vi "Configure Timer Interval Error Filter.vi"(0 "VISA resource name":refnum<visa-resource-name>, 1 "Enable TIE Filter (F: Disable)":bool, 5 "TIE Filter Stopping Frequency (1.5E+6 Hz)":dbl=1500000.0, 7 "TIE Filter Starting Frequency (15000 Hz)":dbl=15000.0, 11 "error in (no error)":errorcluster) -> (4 "VISA resource name out":refnum<visa-resource-name>, 15 "error out":errorcluster)   [LabVIEW 2013, in "Agilent 90000 Series.lvlib"]
doc: "Configures the timer interval error filter characteristics."
uses:
  Agilent 90000 Series.lvlib
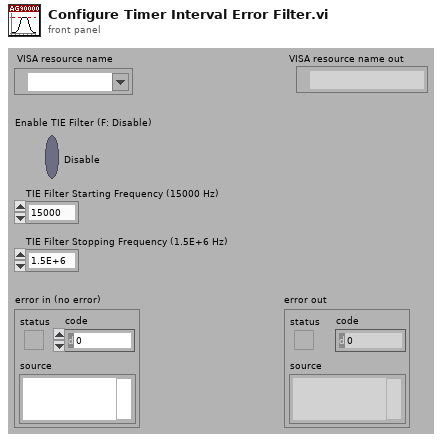
[diagram p1: front panel]
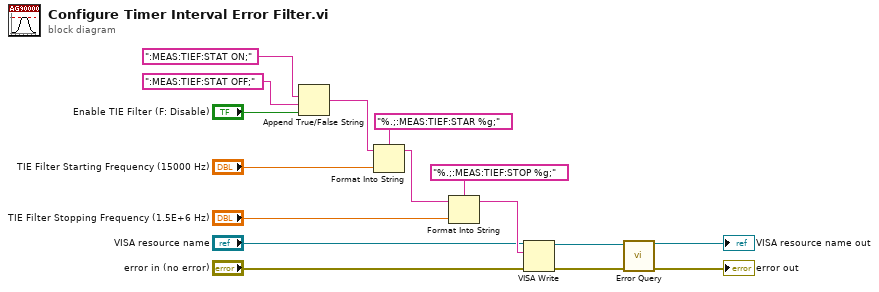
[diagram p0: block diagram]
diagram:
  n1 = Append True/False String(1:"Enable TIE Filter (F: Disable)", 2:":MEAS:TIEF:STAT OFF;", 3:":MEAS:TIEF:STAT ON;") -> (0:w13:string)  [unwired: 1 out]
  n2 = Format Into String(format string="%.;:MEAS:TIEF:STAR %g;", initial string=w13, "TIE Filter Starting Frequency (15000 Hz)") -> (resulting string=w10:string)  [unwired: 1 in, 1 out]
  n3 = Format Into String(format string="%.;:MEAS:TIEF:STOP %g;", initial string=w10, "TIE Filter Stopping Frequency (1.5E+6 Hz)") -> (resulting string=w7:string)  [unwired: 1 in, 1 out]
  n4 = VISA Write(VISA resource name="VISA resource name", write buffer=w7, error in (no error)="error in (no error)") -> (VISA resource name out=w4:refnum<visa-resource-name>, error out=w3:errorcluster)  [unwired: 1 out]
  n5 = call "Error Query.vi"("error in (no error)"=w3, "VISA resource name"=w4) -> ("error out"=→"error out":errorcluster, "VISA resource name out"=→"VISA resource name out":refnum<visa-resource-name>)  [unwired: 8 out]
